vi "Fetch.vi"(8 "error in (no error)":errorcluster, 10 "Message in":refnum<class "FetchMessage.lvclass">, 11 "Test_ExampleClassA in":refnum<class "Test_ExampleClassA.lvclass">) -> (0 "error out":errorcluster, 3 "Test_ExampleClassA out":refnum<class "Test_ExampleClassA.lvclass">)   [LabVIEW 2012, in "Test_ExampleClassA.lvclass"]
doc: "Fetches data received from the test subject (that acts as observee)."
uses:
  Test_ExampleClassA.lvclass
  FetchMessage/FetchMessage.lvclass
  MurmexTest/MurmexTest.lvclass
  Test_ExampleClassA.lvclass/Test_ExampleClassA.ctl
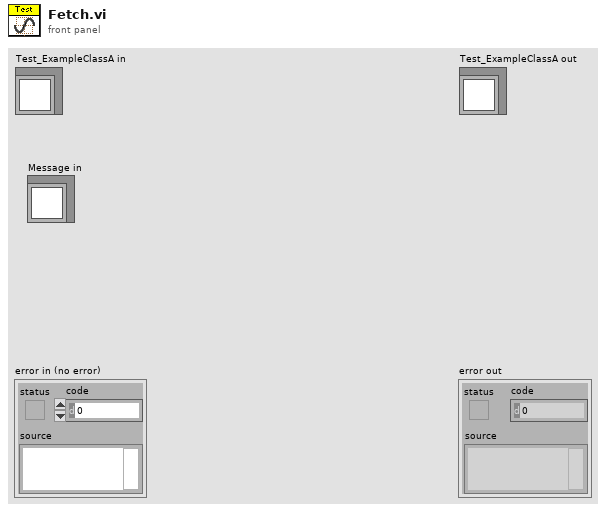
[diagram p1: front panel]
types:
  T1 = typedef "Murmex.lvlib/FetchMessage.lvclass/Channel data cluster.ctl" = cluster{"channel id":i32, "data UInt8":u8[], "data type":T2, "dimensions":i32[], "physical units":T3[], "waveform dt":dbl, "waveform":T4}
  T2 = typedef "Murmex.lvlib/Murmex.lvclass/data_type_enum.ctl" = enum16{"Float128", "Float64", "Float32", "Int64", "Int32", "Int16", "Int8", "UInt64", "UInt32", "UInt16", "UInt8", "Boolean", "String"}
  T3 = typedef "Physical Units__ogtk.ctl" = cluster{"Base Units":enum16{"radian", "steradian", "second", "meter", "kilogram", "ampere", "kelvin", "mole", "candela"}, "Exponent":i16}
  T4 = typedef "waveform_type_enum.ctl" = enum16{"no waveform", "analog", "digital"}
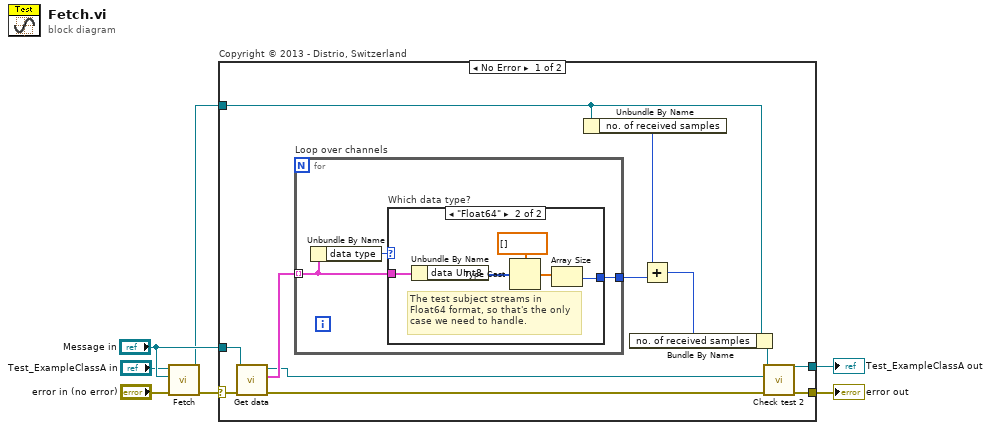
[diagram p0: block diagram]
diagram:
  n1 = call-parent "Fetch.vi"("error in (no error)"="error in (no error)", "Message in"="Message in", "Murmex in"="Test_ExampleClassA in") -> ("error out"=w3:errorcluster, "Murmex out"=w1:refnum<class "Test_ExampleClassA.lvclass">)  [unwired: 7 in]
  n2 = case "Copyright © 2013 - Distrio, Switzerland" shown="No Error" w3 {
    selector: w3 -> [w19 w29]
    tunnel: [w17 w29] -> w7
    tunnel: [w15 w28] -> w6
    tunnel: "Message in" -> [w10 _]
    tunnel: w1 -> [w11 w28]
    frame No Error {
      n3 = call "Get data.vi"("error in (no error)"=w19, "FetchMessage.lvclass"=w10) -> ("error out"=w13:errorcluster, "data (channels)"=w18:T1[], "FetchMessage out"=w9:refnum<class "FetchMessage.lvclass">)  [unwired: 7 in]
      n4 = for "Loop over channels" {
        tunnel: w18 -> [w21] mode=indexing
        tunnel: [w22] -> w12
        n5 = Unbundle By Name(w21) -> ("data type"=w20:T2)
        n6 = case "Which data type?" shown="\"Float64\"" w20 {
          tunnel: w21 -> [_ w24]
          tunnel: [_ w25] -> w22
          frame "Float128", Default {
          }
          frame "Float64" {
            # "The test subject streams in Float64 format, so that's the only case we need to handle."
            n7 = Unbundle By Name(w24) -> ("data UInt8"=w23:u8[])
            n8 = Type Cast(type=dbl[] [] ("data (UInt8)"), x=w23) -> (*(type *) &x=w26:dbl[])
            n9 = Array Size(array=w26) -> (size(s)=w25:i32)
          }
        }
      }
      n10 = Unbundle By Name(w11) -> ("no. of received samples"=w8:i32)
      n11 = Add(x=w8, y=w12) -> (x+y=w14:i32)
      n12 = Bundle By Name(cluster=w11, "no. of received samples"=w14) -> (w16:refnum<class "Test_ExampleClassA.lvclass">)
      n13 = call "Check test 2.vi"("error in (no error)"=w13, "Message in"=w9, "Test_ExampleClassA in"=w16) -> ("error out"=w17:errorcluster, "Test_ExampleClassA out"=w15:refnum<class "Test_ExampleClassA.lvclass">)  [unwired: 7 in]
    }
    frame Error {
    }
  }
  "error out" <- w7
  "Test_ExampleClassA out" <- w6
